vi "ShowPanelRequest.vi"(8 "error in (no error)":errorcluster, 10 "ShowPanel?":bool, 11 "ModuleID":i32=-1) -> (0 "error out":errorcluster)   [LabVIEW 2018, in "DigitizerModule.lvlib"]
uses:
  DigitizerModule.lvlib
  DigitizerShared/clEventType.ctl
  <vilib>/Utility/error.llb/Error Cluster From Error Code.vi
  <vilib>/ErrorRing/Error Ring.xnode
  DigitizerShared/DigitizerShared.lvlib
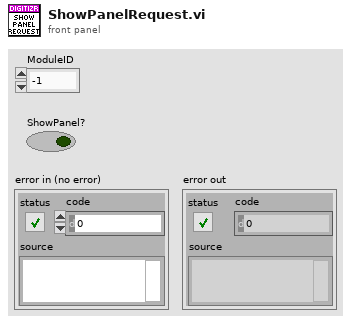
[diagram p1: front panel]
types:
  T1 = typedef "DigitizerShared.lvlib/clRequestEvents.ctl" = cluster{"StopRequest":refnum<user-event>, "PathToINI":refnum<user-event>, " LoadPlugin":refnum<user-event>, "ShowPanel":refnum<user-event>, "PrefDlg":refnum<user-event>, "ReadChannels":refnum<user-event>, "WriteChannels":refnum<user-event>, "ConfigChannels":refnum<user-event>, "ReadAcq":refnum<user-event>, "WriteAcq":refnum<user-event>, "ConfigAcq":refnum<user-event>, "ReadTriggers":refnum<user-event>, "WriteTriggers":refnum<user-event>, "ConfigTriggers":refnum<user-event>, "FetchWfrm":refnum<user-event>, "ReadWfrm":refnum<user-event>, "Initialize":refnum<user-event>, "Abort":refnum<user-event>, "ReadSyncInfo":refnum<user-event>, "WriteSyncInfo":refnum<user-event>, "Close":refnum<user-event>}
  T2 = typedef "DigitizerShared.lvlib/clEventType.ctl" = cluster{"ModuleID":i32, "Data":variant}
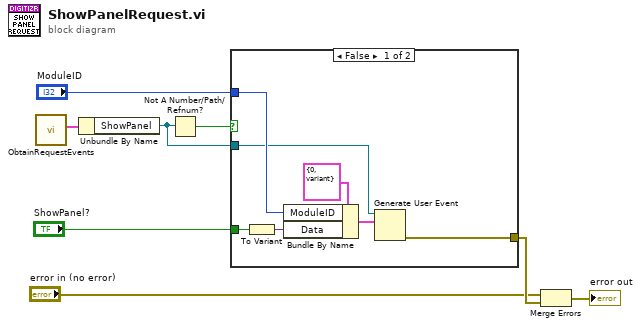
[diagram p0: block diagram]
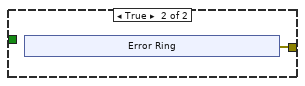
[diagram p2: hidden frame]
diagram:
  n1 = call "ObtainRequestEvents.vi"() -> ("clDigitizerRequestEvents"=w8:T1)  [unwired: 10 in, 1 out]
  n2 = Unbundle By Name(w8) -> ("ShowPanel"=w6:refnum<user-event>)
  n3 = Not A Number/Path/Refnum?(number/path/refnum=w6) -> (NaN/Path/Refnum?=w7:bool)
  n4 = case shown="False" w7 {
    tunnel: w6 -> [w11 _]
    tunnel: "ModuleID" -> [w14 _]
    tunnel: "ShowPanel?" -> [w10 _]
    tunnel: [w9 w16] -> w3
    frame False {
      n5 = To Variant(anything=w10) -> (Variant=w13:variant)
      n6 = Bundle By Name(cluster=T2 {"ModuleID"=0, "Data"=variant} ("clEventType"), "ModuleID"=w14, "Data"=w13) -> (w12:T2)
      n7 = Generate User Event(user event=w11, event data cluster=w12) -> (error out=w9:errorcluster)  [unwired: 2 in, 1 out]
    }
    frame True {
      n8 = xnode "Error Ring"() -> ("error out"=w16:errorcluster)
    }
  }
  n9 = Merge Errors("error in (no error)", w3) -> (→"error out":errorcluster)
